vi "H5Aread_ModifyCode.vi"(0 "XRef":T18, 1 "Terms":T15, 2 "Diagram":T14, 3 "State In":T1) -> (14 "Generated Code?":T8, 15 "Reply":T13, 16 "State Out":T1)   [LabVIEW 2017, in "H5Aread.xnode"]
doc: "This ability VI is called when it is time to define the execution behavior of your XNode via LabVIEW's scripting API. This VI is only called when you have previously informed LabVIEW that you need to script through a ModifyCode reply. Diagram is a reference to a diagram with your VI's current code (generated from the previous GenerateCode or ModifyCode call). This diagram contains exactly one front panel terminal for each terminal of your XNode. Terms is an array of pairs of Term IDs and terminal references. LabVIEW will copy code scripted into this diagram into your XNode and connect everything to the correct terminals. The front panel terminals that are on this diagram are special in that they can only be on the top level diagram.\n \n Generate Code? is used to tell LabVIEW whether or not you want to copy the scripted diagram over. If there is an error and you wish not to commit the changes, then the old XNode behavior will be left unchanged. If you set Generate Code? to false, then GenerateCode will be called next time type propagation is run. Otherwise, GenerateCode or ModifyCode will not be called until you indicate that it should be through the reply on another ability VI.\n \n Because the diagram you are scripting into is separate from the VI containing the XNode instance, type propagation and the data manager will run on the temporary VI after each scripting call.\n \n You should not use the Copy scripting method to move code into the temporary VI. This will adversely affect the user's clipboard. You should use the Move scripting method instead.\n\nDefault behavior: None.\n\nThis ability does not provide UI and OS messages are not handled.\n\nSee also: GenerateCode"
uses:
  <vilib>/UPVI/lvhdf5/attribute.llb/H5Aread.xnode
  <vilib>/XNodeSupport/XNodeXNodeRef.ctl
  <vilib>/XNodeSupport/XNodeTermIDPairs.ctl
  <vilib>/XNodeSupport/XNodeTermIDPair.ctl
  <vilib>/XNodeSupport/XNodeTermRef.ctl
  <vilib>/XNodeSupport/XNodeString.ctl
  <vilib>/XNodeSupport/XNodeTopLevelDiagramRef.ctl
  <vilib>/UPVI/lvhdf5/attribute.llb/H5Aread/H5Aread_State.ctl
  <vilib>/UPVI/lvhdf5/xnodehelpers/TermsPlus.ctl
  <vilib>/XNodeSupport/XNodeTerm3.ctl
  <vilib>/XNodeSupport/XNodeVariant.ctl
  <vilib>/XNodeSupport/XNodeRect32.ctl
  <vilib>/XNodeSupport/XNodeInt.ctl
  <vilib>/XNodeSupport/XNodeBool.ctl
  <vilib>/XNodeSupport/XNodeTermDirection.ctl
  <vilib>/UPVI/lvhdf5/xnodehelpers/TermBehavior.ctl
  <vilib>/XNodeSupport/XNodeError3Array.ctl
  <vilib>/XNodeSupport/XNodeError3.ctl
  <vilib>/XNodeSupport/XNodeStringArray.ctl
  <vilib>/XNodeSupport/NI_XNodeSupport.lvlib
panel:
  in  "vi path":path
  # "LVHDF5 Toolkit\nCopyright (c) 2005-2013 by Jason D. Sommerville\nCopyright (c) 2014 by UPVI, LLC.\n\nThis use and distribution of this file is governed by the terms found in \nLICENSE.txt distributed with this toolkit and installed at\n <user.lib>\\_lvhdf5\\LICENSE.txt"
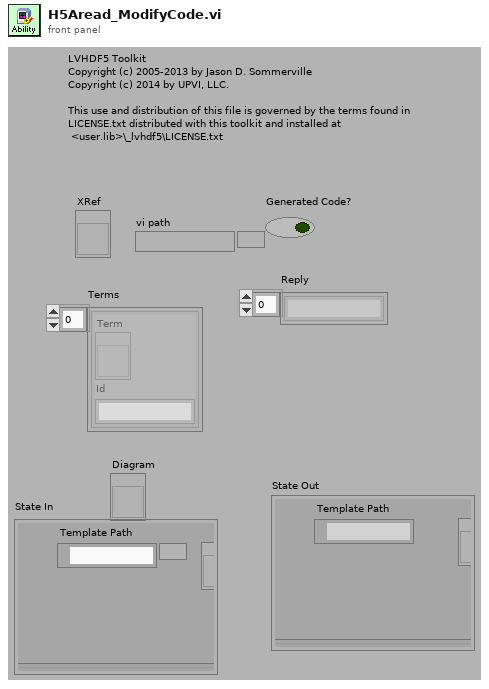
[diagram p1: front panel]
types:
  T1 = typedef "H5Aread.xnode/H5Aread_State.ctl" = cluster{"Template Path":path, "Template Ref":refnum<vi>, "Terms":T2[], "Display Name":string, "Image":picture, "Errors":T11, "Generated?":bool}
  T2 = typedef "TermsPlus.ctl" = cluster{"Term 3":T3, "Default Type":variant, "Behavior":T10, "Behavior Arg":string, "WiredResponse":bool, "Wired":enum16{"Unknown", "Unwired", "Wired"}}
  T3 = typedef "NI_XNodeSupport.lvlib/XNodeTerm3.ctl" = cluster{"Name":T4, "Id":T4, "Type":T5, "Bounds":T6, "Input?":T8, "Required?":T8, "Recommended?":T8, "Adaptive?":T8, "Hidden?":T8, "Direction":T9, "Break Wire?":T8}
  T4 = typedef "NI_XNodeSupport.lvlib/XNodeString.ctl" = string
  T5 = typedef "NI_XNodeSupport.lvlib/XNodeVariant.ctl" = variant
  T6 = typedef "NI_XNodeSupport.lvlib/XNodeRect32.ctl" = cluster{"Left":T7, "Top":T7, "Right":T7, "Bottom":T7}
  T7 = typedef "NI_XNodeSupport.lvlib/XNodeInt.ctl" = i32
  T8 = typedef "NI_XNodeSupport.lvlib/XNodeBool.ctl" = bool
  T9 = typedef "NI_XNodeSupport.lvlib/XNodeTermDirection.ctl" = enum32{"Auto", "Up", "Down", "Left", "Right", "Center"}
  T10 = typedef "TermBehavior.ctl" = enum16{"Normal", "Anything", "LVType", "Path or Ref", "Attr Name", "Attr Poly", "Elt Poly", "Dset Poly", "WDT Poly"}
  T11 = typedef "NI_XNodeSupport.lvlib/XNodeError3Array.ctl" = T12[]
  T12 = typedef "NI_XNodeSupport.lvlib/XNodeError3.ctl" = cluster{"Error":T4, "Details":T4, "Help File":T4, "Help Topic":T4}
  T13 = typedef "NI_XNodeSupport.lvlib/XNodeStringArray.ctl" = T4[]
  T14 = typedef "NI_XNodeSupport.lvlib/XNodeTopLevelDiagramRef.ctl" = refnum<vi>
  T15 = typedef "NI_XNodeSupport.lvlib/XNodeTermIDPairs.ctl" = T16[]
  T16 = typedef "NI_XNodeSupport.lvlib/XNodeTermIDPair.ctl" = cluster{"Term":T17, "Id":T4}
  T17 = typedef "NI_XNodeSupport.lvlib/XNodeTermRef.ctl" = refnum<vi>
  T18 = typedef "NI_XNodeSupport.lvlib/XNodeXNodeRef.ctl" = refnum<vi>
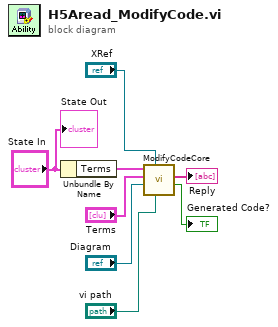
[diagram p0: block diagram]
diagram:
  n1 = Unbundle By Name("State In") -> ("Terms"=w2:T2[])
  n2 = call <vilib>:"ModifyCodeCore.vi"("vi path (for debug)"="vi path", "XNode in"="XRef", "Diagram"="Diagram", "Terms"="Terms", "State Terms"=w2) -> ("Generated Code?"=→"Generated Code?":T8, "Reply"=→"Reply":T13)  [unwired: 5 in]
  "State Out" <- "State In"
